vi "Split num query command.vi"(0 "System no.":i32=1 min=1 max=4 step=1, 1 "Query command":u16(ring) items=["POS?", "MOV?", "VOL?", "SVA?"], 2 "Axes to query":string[](array[string]), 5 "error in":errorcluster) -> (14 "Values":dbl[](array[numeric]) format="%.6f", 19 "error out":errorcluster)   [LabVIEW 2020]
doc: "Splits numerical query command with more than one axis specification into the corresponding one-axis commands and returns answers for all given axes. Supported commands are POS?, MOV?, VOL?, SVA? (more commands can be added).\nOld command. Use Split multiple axes command.vi instead."
panel:
  # "Splits numerical query command with more than one axis specification\n into the corresponding one-axis commands and\nreturns answers for all given axes. Supported commands are POS?, MOV?, \nVOL?, SVA? (more commands can be added). \nOld command. Use Split multiple axes command.vi instead."
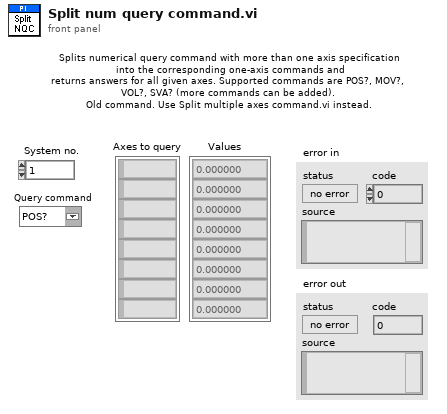
[diagram p1: front panel]
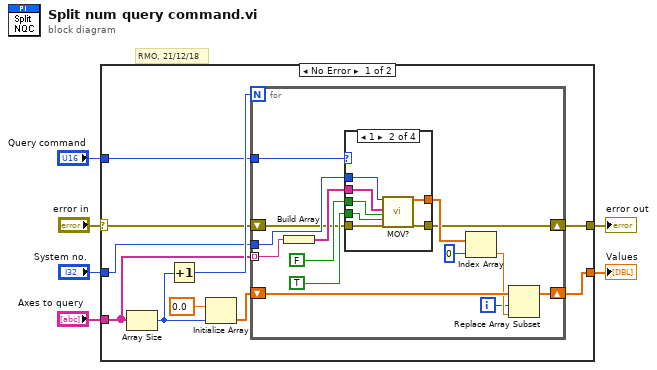
[diagram p0: block diagram]
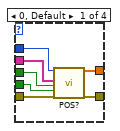
[diagram p2: hidden frame]
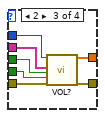
[diagram p3: hidden frame]
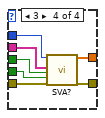
[diagram p4: hidden frame]
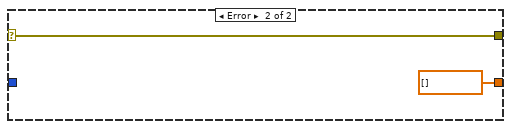
[diagram p5: hidden frame]
diagram:
  # "RMO, 21/12/18"
  n1 = case shown="No Error" "error in" {
    selector: "error in" -> [w7 w59]
    tunnel: "Query command" -> [w12 _]
    tunnel: "Axes to query" -> [w11 _]
    tunnel: "System no." -> [w10 _]
    tunnel: [w9 dbl[] []] -> w3
    tunnel: [w8 w59] -> w2
    frame No Error {
      n2 = Array Size(array=w11) -> (size(s)=w14:i32)
      n3 = Increment(x=w14) -> (x+1=w13:i32)
      n4 = Initialize Array(0.0, w14) -> (w15:dbl[])
      n5 = for {
        N: w13 -> [_]
        tunnel: w11 -> [w23] mode=indexing
        tunnel: w10 -> [w30]
        shift-right: [w25] -> w9
        shift-left: w15 -> [w28]
        tunnel: w12 -> [w24]
        shift-right: [w18] -> w8
        shift-left: w7 -> [w17]
        i -> [w20]
        n6 = Build Array(w23) -> (w29:string[])
        n7 = case shown="1" w24 {
          tunnel: w17 -> [w37 w42 w49 w56]
          tunnel: w30 -> [w36 w44 w51 w58]
          tunnel: [w35 w41 w48 w55] -> w18
          tunnel: w29 -> [w34 w43 w50 w57]
          tunnel: [w33 w40 w47 w54] -> w27
          tunnel: FALSE ("All axes?") -> [w32 w39 w46 w53]
          tunnel: TRUE ("Axis identifier?") -> [w31 w38 w45 w52]
          frame 0, Default {
            n8 = call "POS?.vi"("System no."=w36, "Axes to query"=w34, "All axes?"=w32, "Axis identifier?"=w31, "error in"=w37) -> ("Position"=w33:dbl[], "error out"=w35:errorcluster)  [unwired: 13 out]
          }
          frame 1 {
            n9 = call "MOV?.vi"("System no."=w44, "Axes to query"=w43, "All axes?"=w39, "Axis identifier?"=w38, "error in"=w42) -> ("Target position"=w40:dbl[], "error out"=w41:errorcluster)  [unwired: 13 out]
          }
          frame 2 {
            n10 = call "VOL?.vi"("System no."=w51, "Axes to query"=w50, "All axes?"=w46, "Axis identifier?"=w45, "error in"=w49) -> ("Current PZT voltage"=w47:dbl[], "error out"=w48:errorcluster)  [unwired: 13 out]
          }
          frame 3 {
            n11 = call "SVA?.vi"("System no."=w58, "Axes to query"=w57, "All axes?"=w53, "Axis identifier?"=w52, "error in"=w56) -> ("Commanded PZT voltage"=w54:dbl[], "error out"=w55:errorcluster)  [unwired: 13 out]
          }
        }
        n12 = Index Array(array=w27, index=0 ("Index")) -> (element=w26:dbl)
        n13 = Replace Array Subset(array=w28, new element=w26, index=w20) -> (w25:dbl[])
      }
    }
    frame Error {
    }
  }
  "error out" <- w2
  "Values" <- w3
